vi "Move Frame Settings.vi"(8 "error in (no error)":errorcluster, 10 "Frames":T4(array[cluster]) {"Frame Transmit Info"."Transmit Time" format="%#_p"}, 11 "Ref in":T1 format="%.0x") -> (0 "error out":errorcluster, 3 "Ref out":T1 format="%.0x")   [LabVIEW 2013, in "J1939 Addon System Explorer.lvlib"]
uses:
  J1939 Addon System Explorer.lvlib
  Shared/Types/XNET Frame Event Properties.ctl
  Shared/Types/SPN Properties.ctl
  <vilib>/NI Veristand/Custom Device API/Custom Device Item Ref.ctl
  <vilib>/NI Veristand/Custom Device API/Custom Device Channel.ctl
  <vilib>/NI Veristand/Custom Device API/Custom Device Channel Type.ctl
  Shared/SubVIs/Constants.vi
  <vilib>/NI Veristand/Custom Device API/Set Item Property (Variant).vi
  Shared/J1939 Addon Shared.lvlib
  <vilib>/NI Veristand/Custom Device API/Custom Device API.lvlib
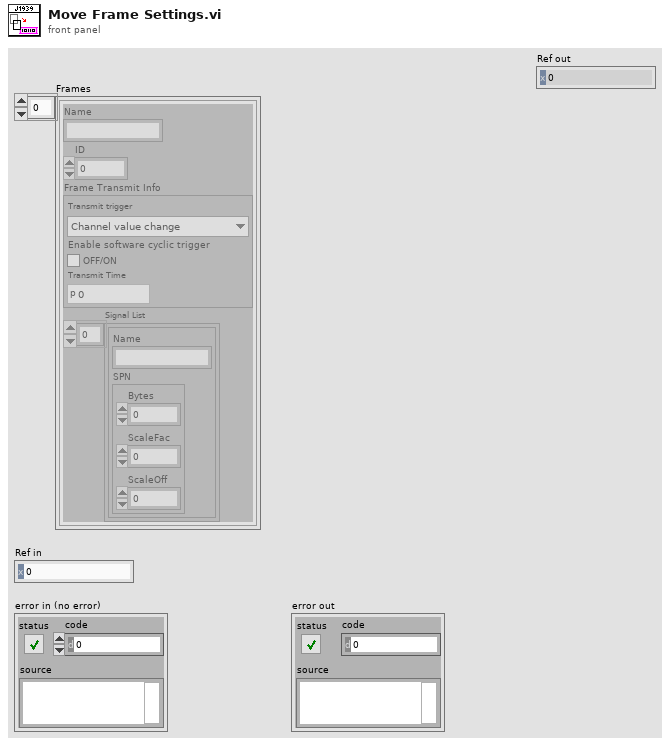
[diagram p1: front panel]
types:
  T1 = typedef "Custom Device API.lvlib/Custom Device Item Ref.ctl" = u64
  T2 = typedef "J1939 Addon Shared.lvlib/XNET Frame Event Properties.ctl" = cluster{"Transmit trigger":enum16{"Channel value change"}, "Enable software cyclic trigger":bool, "Transmit Time":dbl}
  T3 = typedef "J1939 Addon Shared.lvlib/SPN Properties.ctl" = cluster{"Bytes":u32, "ScaleFac":dbl, "ScaleOff":dbl}
  T4 = cluster{"Name":string, "ID":u32, "Frame Transmit Info":T2, "Signal List":cluster{"Name":string, "SPN":T3}[]}[]
  T5 = typedef "Custom Device API.lvlib/Custom Device Item Info.ctl" = cluster{"Name":string, "Is Channel":bool, "GUID":string, "Is Waveform":bool}
  T6 = typedef "Custom Device API.lvlib/Custom Device Channel.ctl" = cluster{"Type":T7, "Units":string, "Default Value":dbl, "Faultable":bool, "Scalable":bool}
  T7 = typedef "Custom Device API.lvlib/Custom Device Channel Type.ctl" = enum16{"Input", "Output"}
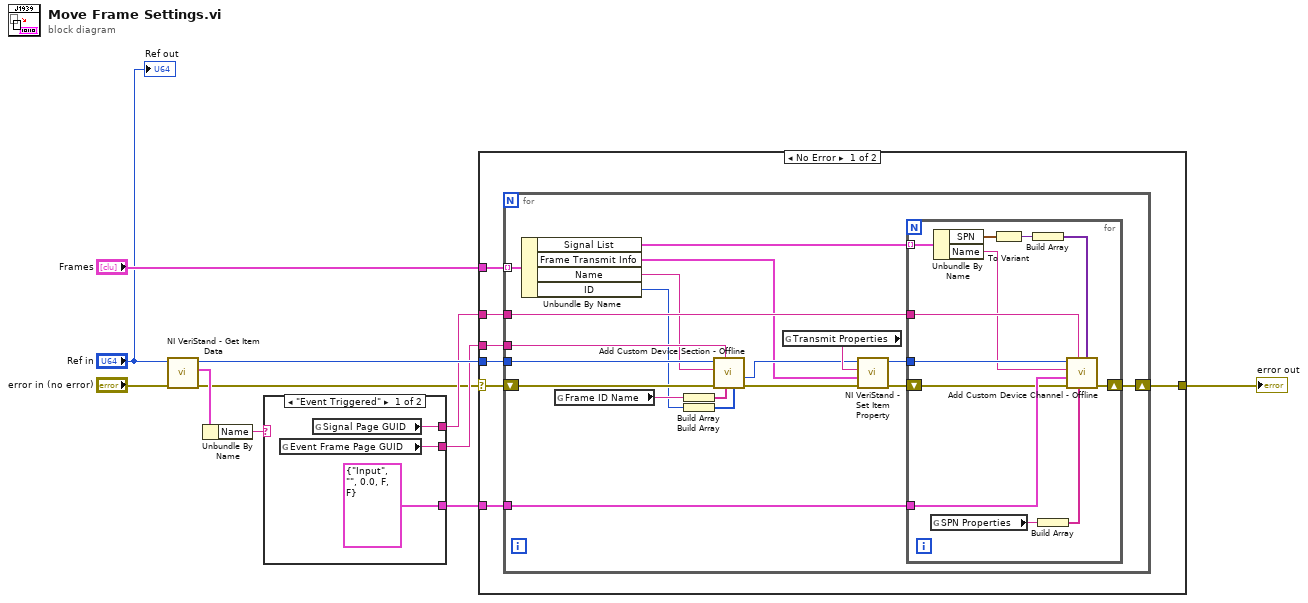
[diagram p0: block diagram]
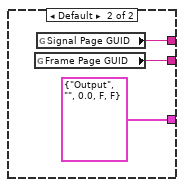
[diagram p2: hidden frame]
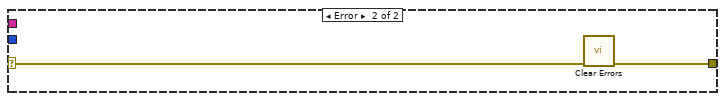
[diagram p3: hidden frame]
diagram:
  n1 = call <vilib>:"NI VeriStand - Get Item Data.vi"("error in (no error)"="error in (no error)", "Item Ref in"="Ref in") -> ("error out"=w1:errorcluster, "Item Info"=w6:T5, "Item Ref out"=w7:T1)  [unwired: 7 out]
  n2 = Unbundle By Name(w6) -> ("Name"=w5:string)
  n3 = case shown="\"Event Triggered\"" w5 {
    tunnel: [w14 w17] -> w4
    tunnel: [w13 w16] -> w3
    tunnel: [T6 {"Type"=enum."Input", "Units"="", "Default Value"=0.0, "Faultable"=FALSE, "Scalable"=FALSE} ("Channel") T6 {"Type"=enum."Output", "Units"="", "Default Value"=0.0, "Faultable"=FALSE, "Scalable"=FALSE} ("Channel")] -> w2
    frame "Event Triggered" {
      n4 = global read "Constants.vi" "Event Frame Page GUID"() -> (w13:string)
      n5 = global read "Constants.vi" "Signal Page GUID"() -> (w14:string)
    }
    frame Default {
      n6 = global read "Constants.vi" "Frame Page GUID"() -> (w16:string)
      n7 = global read "Constants.vi" "Signal Page GUID"() -> (w17:string)
    }
  }
  n8 = case shown="No Error" w1 {
    selector: w1 -> [w22 w57]
    tunnel: [w24 w56] -> w8
    tunnel: w7 -> [w23 _]
    tunnel: w4 -> [w21 _]
    tunnel: w3 -> [w20 _]
    tunnel: w2 -> [w19 _]
    tunnel: "Frames" -> [w18 _]
    frame No Error {
      n9 = for {
        shift-right: [w43] -> w24
        shift-left: w22 -> [w28]
        tunnel: w23 -> [w42]
        tunnel: w21 -> [w40]
        tunnel: w20 -> [w39]
        tunnel: w19 -> [w37]
        tunnel: w18 -> [w29] mode=indexing
        n10 = Unbundle By Name(w29) -> ("Signal List"=w30:cluster{"Name":string, "SPN":T3}[], "Frame Transmit Info"=w27:T2, "Name"=w25:string, "ID"=w26:u32)
        n11 = global read "Constants.vi" "Frame ID Name"() -> (w41:string)
        n12 = Build Array(w41) -> (w33:string[])
        n13 = Build Array(w26) -> (w34:u32[])
        n14 = call "Add Custom Device Section - Offline.vi"("Property Values"=w34, "Property names"=w33, "GUID (Default Section)"=w39, "error in (no error)"=w28, "Section Name"=w25, "Parent Ref in"=w42) -> ("error out"=w32:errorcluster, "Section Ptr"=w31:T1)  [unwired: 2 in, 2 out]
        n15 = global read "Constants.vi" "Transmit Properties"() -> (w38:string)
        n16 = call-poly <vilib>:"NI VeriStand - Set Item Property.vi"("error in (no error)"=w32, "Value"=w27, "Property Name"=w38, "Item Ref in"=w31) -> ("error out"=w36:errorcluster, "Item Ref out"=w35:T1)  [unwired: 5 in, 1 out]
        n17 = for {
          tunnel: w40 -> [w54]
          tunnel: w37 -> [w53]
          tunnel: w35 -> [w51]
          shift-right: [w55] -> w43
          shift-left: w36 -> [w52]
          tunnel: w30 -> [w50] mode=indexing
          n18 = global read "Constants.vi" "SPN Properties"() -> (w45:string)
          n19 = Unbundle By Name(w50) -> ("SPN"=w49:T3, "Name"=w46:string)
          n20 = To Variant(anything=w49) -> (Variant=w48:variant)
          n21 = Build Array(w48) -> (w47:variant[])
          n22 = Build Array(w45) -> (w44:string[])
          n23 = call "Add Custom Device Channel - Offline.vi"("Property Values"=w47, "Property names"=w44, "GUID (Default Channel)"=w54, "error in (no error)"=w52, "Channel"=w53, "Channel Name"=w46, "Parent Ref in"=w51) -> ("error out"=w55:errorcluster)  [unwired: 1 in, 3 out]
        }
      }
    }
    frame Error {
      n24 = call <vilib>:"Clear Errors.vi"("error in (no error)"=w57) -> ("error out"=w56:errorcluster)  [unwired: 6 in]
    }
  }
  "error out" <- w8
  "Ref out" <- "Ref in"
